vi "Send Remote Request.vi"(5 "Target Task (None)":string, 6 "Timeout mS (5000)":i32=5000, 7 "Target Node":string, 8 "error in (no error)":errorcluster, 9 "Message Type":string, 10 "Message":refnum<class "Message.lvclass">, 11 "Module in":refnum<class "Module.lvclass">) -> (0 "error out":errorcluster, 2 "Reply":T1, 3 "Module out":refnum<class "Module.lvclass">)   [LabVIEW 2020, in "Volatus.lvlib" / "Module.lvclass"]
uses:
  Module.lvclass
  lv-protoc/LV-Proto/Message/Message.lvclass
  messages/TcpPayload/Data.ctl
  Module.lvclass/Module.ctl
  VolatusAPI/VolatusAPI.lvclass
  messages/TcpPayload/TcpPayload.lvlib
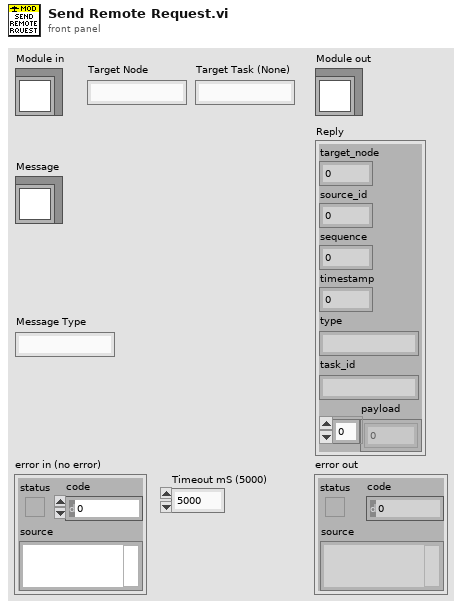
[diagram p1: front panel]
types:
  T1 = typedef "TcpPayload.lvlib/Data.ctl" = cluster{"target_node":u32, "source_id":u32, "sequence":u32, "timestamp":i64, "type":string, "task_id":string, "payload":u8[]}
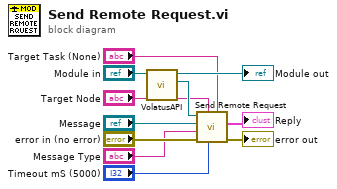
[diagram p0: block diagram]
diagram:
  n1 = call "VolatusAPI.vi"("Module in"="Module in") -> ("VolatusAPI"=w9:refnum<class "VolatusAPI.lvclass">, "Module out"=→"Module out":refnum<class "Module.lvclass">)  [unwired: 9 in]
  n2 = call "Send Remote Request.vi"("Target Task (None)"="Target Task (None)", "Timeout mS (5000)"="Timeout mS (5000)", "Target Name"="Target Node", "error in (no error)"="error in (no error)", "Message Type"="Message Type", "Message"="Message", "VolatusAPI in"=w9) -> ("error out"=→"error out":errorcluster, "Reply"=→"Reply":T1)  [unwired: 2 in, 1 out]
